vi "Bus Interface.vi"(0 "Basecard Config Registers":refnum<class "7902R Basecard Config Registers.lvclass">, 1 "abort":bool, 5 "instruction":T2, 9 "input valid":bool) -> (6 "response":T1, 10 "done":bool, 14 "ready for input":bool)   [LabVIEW 2019, in "7902R Basecard Config Registers.lvclass"]
uses:
  7902R Basecard Config Registers.lvclass
  <vilib>/eio/EIOMethodNode/EIOMethodNode.xnode
  <instrlib>/_niInstr/Instruction Framework/v1/FPGA/Typedefs/niInstr Instruction Framework v1 FPGA.lvlib
  <vilib>/rvi/eio/common/nirviEmuTemplateMethod_errors.vi
  <instrlib>/_niInstr/Instruction Framework/v1/FPGA/Interfaces/Address Space/Address Space Instruction.ctl
  <instrlib>/_niInstr/Instruction Framework/v1/FPGA/Interfaces/Address Space/Address Space.lvclass
  <instrlib>/_niInstr/Instruction Framework/v1/FPGA/Typedefs/Response.ctl
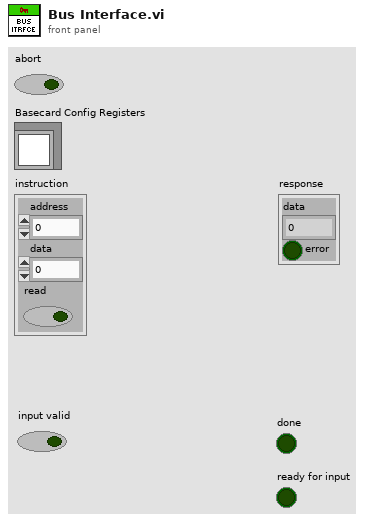
[diagram p1: front panel]
types:
  T1 = typedef "niInstr Instruction Framework v1 FPGA.lvlib/Response.ctl" = cluster{"data":u64, "error":bool}
  T2 = typedef "niInstr Instruction Framework Interfaces v1 FPGA.lvlib/Address Space.lvclass/Address Space Instruction.ctl" = cluster{"address":u32, "data":u64, "read":bool}
  T3 = cluster{"register read data":u64, "register read data valid":bool, "registers ready":bool}
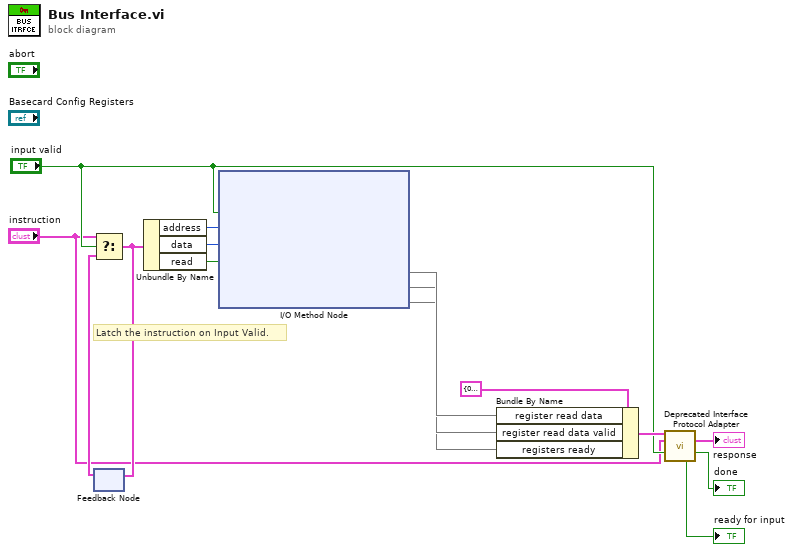
[diagram p0: block diagram]
diagram:
  # "Latch the instruction on Input Valid."
  n1 = feedback #1() -> (w14:T2)  [unwired: 1 in]
  n2 = Select(t="instruction", s="input valid", f=w14) -> (s? t:f=w15:T2)
  n3 = feedback-in #1(w15) -> ()
  n4 = Unbundle By Name(w15) -> ("address"=w13:u32, "data"=w12:u64, "read"=w11:bool)
  n5 = xnode "I/O Method Node"("Input Valid"="input valid", "Address"=w13, "Data In"=w12, "Read"=w11) -> ("Data Out"=w8, "Output Valid"=w7, "Ready for Input"=w6)  [unwired: 1 in, 1 out]
  n6 = Bundle By Name(cluster=T3 {"register read data"=0, "register read data valid"=FALSE, "registers ready"=FALSE} ("register output"), "register read data"=w8, "register read data valid"=w7, "registers ready"=w6) -> (w10:T3)
  n7 = call <instrlib>:"Deprecated Interface Protocol Adapter.vi"("register output"=w10, "instruction"="instruction", "input valid (instruction)"="input valid") -> ("response data"=→"response":T1, "output valid (response)"=→"done":bool, "ready for input"=→"ready for input":bool)  [unwired: 10 in]
